vi "VectorCased.vi"(11 "XYUVArray":dbl[][](array[numeric])=[[-138.0, 28.0, -5.0, -3.0], [-92.0, 28.0, -10.0, -5.5], [-46.0, 28.0, -5.0, -10.5], [0.0, 28.0, -9.0, 3.5], [46.0, 28.0, -22.0, 1.0], [92.0, 28.0, -24.5, -9.0], [138.0, 28.0, -16.0, -23.0], [-138.0, 60.0, -6.0, -2.0], [-92.0, 60.0, -7.0, -12.0], [-46.0, 60.0, -6.0, -11.0], [0.0, 60.0, -9.0, 3.0], [46.0, 60.0, -5.5, 6.0], [92.0, 60.0, -10.0, -7.5], [138.0, 60.0, -17.0, -22.0], [-138.0, 92.0, 0.5, 2.0], [-92.0, 92.0, -1.5, -15.0], [-46.0, 92.0, -1.5, -10.5], [0.0, 92.0, 1.0, -1.5], [46.0, 92.0, 1.0, 3.0], [92.0, 92.0, -2.5, -7.5], [138.0, 92.0, -5.0, -17.0], [-138.0, 124.0, 18.5, 15.0], [-92.0, 124.0, 10.5, -2.5], [-46.0, 124.0, 6.5, -2.0], [0.0, 124.0, 7.5, 5.0], [46.0, 124.0, 9.5, 12.5], [92.0, 124.0, 14.0, 8.5], [138.0, 124.0, 6.5, -4.0], [-138.0, 156.0, 13.5, 14.5], [-92.0, 156.0, 19.5, 4.0], [-46.0, 156.0, 12.5, -1.0], [0.0, 156.0, 10.5, 3.5], [46.0, 156.0, 14.0, 11.0], [92.0, 156.0, 17.5, 10.5], [138.0, 156.0, 12.0, -4.5], [-138.0, 188.0, 9.0, 16.5], [-92.0, 188.0, 10.0, 8.0], [-46.0, 188.0, 14.0, 4.0], [0.0, 188.0, 15.5, 8.0], [46.0, 188.0, 14.5, 11.0], [92.0, 188.0, 21.5, 11.0], [138.0, 188.0, 19.0, 0.5], [-138.0, 214.0, 12.5, 11.5], [-92.0, 214.0, 17.5, 6.0], [-46.0, 214.0, 17.0, 9.5], [0.0, 214.0, 14.5, 10.5], [46.0, 214.0, 19.0, 10.5], [92.0, 214.0, 20.0, 7.0], [138.0, 214.0, 16.5, 7.0]]) -> ()   [LabVIEW 2010]
panel:
  in  "ArrowScale":dbl(slide)=0.3 min=0.0 step=0.1 scale=0.0..0.5
  in  "stop":bool
  in  "Border":dbl(slide)=0.2 min=0.0 step=0.05 scale=0.0..0.2
  in  "VectorScale":dbl(slide)=1.5 min=0.0 step=0.25 scale=0.0..10.0
  out "VectorPicture":picture
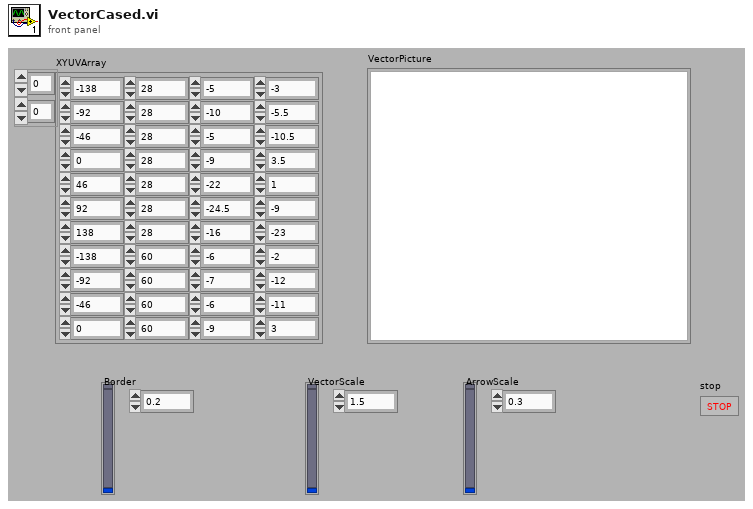
[diagram p1: front panel]
types:
  T1 = typedef "LVBoundsTypeDef.ctl" = cluster{"Width":u32, "Height":u32}
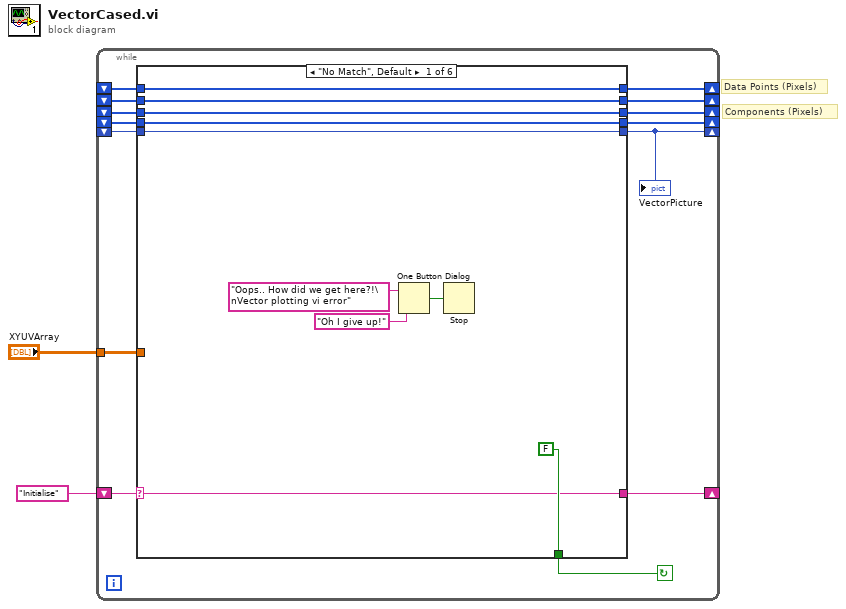
[diagram p0: block diagram]
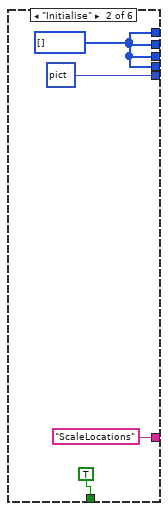
[diagram p2: hidden frame]
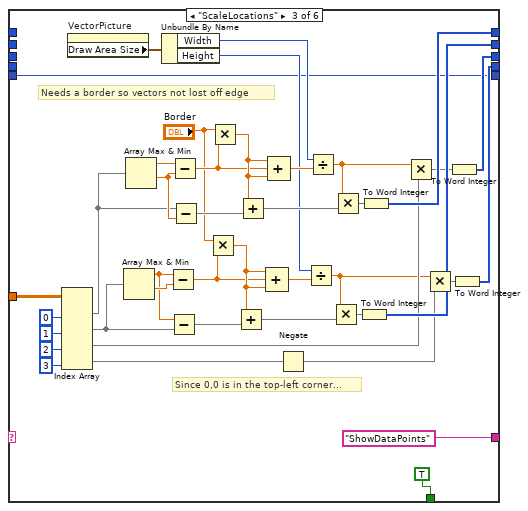
[diagram p3: hidden frame]
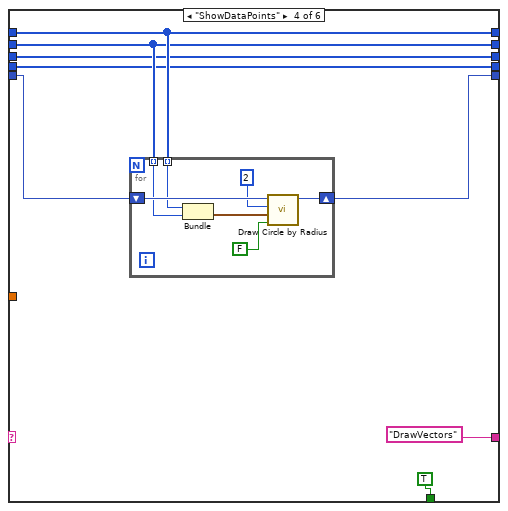
[diagram p4: hidden frame]
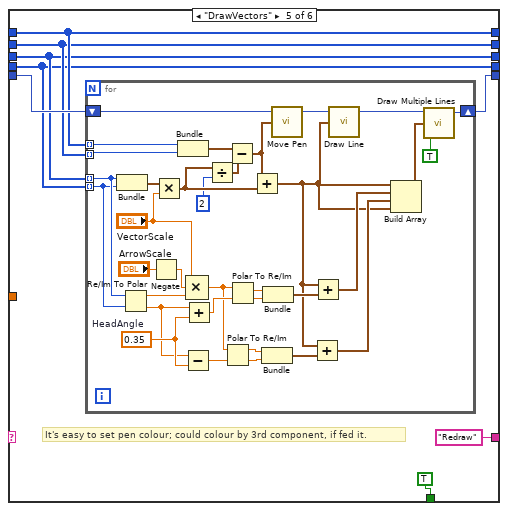
[diagram p5: hidden frame]
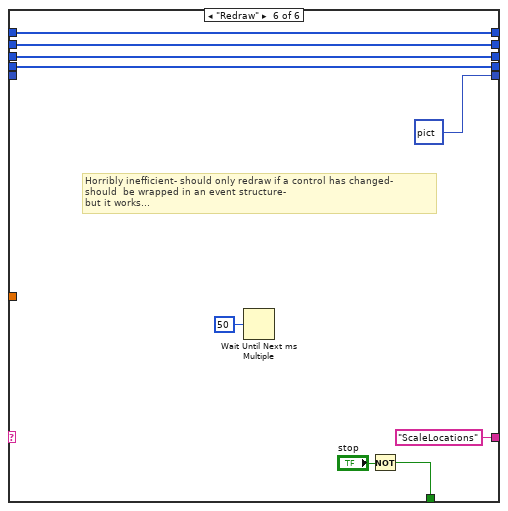
[diagram p6: hidden frame]
diagram:
  # "Components (Pixels)"
  # "Data Points (Pixels)"
  n1 = while {
    shift-right: [w12] -> _
    shift-left: "Initialise" -> [w16]
    shift-right: [w7] -> _
    shift-left: _ -> [w14]
    tunnel: "XYUVArray" -> [w13]
    shift-right: [w11] -> _
    shift-left: _ -> [w9]
    shift-right: [w10] -> _
    shift-left: _ -> [w8]
    shift-right: [w6] -> _
    shift-left: _ -> [w4]
    shift-right: [w5] -> _
    shift-left: _ -> [w3]
    stop <- w15 continue-if-true
    n2 = case shown="\"No Match\", Default" w16 {
      selector: w16 -> [w25 _ _ _ _ _]
      tunnel: [FALSE TRUE TRUE TRUE TRUE w131] -> w15
      tunnel: [w24 picture data[5B] ("new picture") w31 w75 w93 picture data[5B] ("new picture")] -> w7
      tunnel: w14 -> [w24 _ w31 w79 w94 _]
      tunnel: w13 -> [_ _ w66 _ _ _]
      tunnel: [w25 "ScaleLocations" "ShowDataPoints" "DrawVectors" "Redraw" "ScaleLocations"] -> w12
      tunnel: [w23 w27 w45 w78 w92 w137] -> w11
      tunnel: [w22 w27 w44 w77 w91 w136] -> w10
      tunnel: w9 -> [w23 _ _ w78 w92 w137]
      tunnel: w8 -> [w22 _ _ w77 w91 w136]
      tunnel: [w21 w27 w34 w74 w90 w135] -> w6
      tunnel: [w20 w27 w33 w73 w89 w134] -> w5
      tunnel: w4 -> [w21 _ _ w74 w90 w135]
      tunnel: w3 -> [w20 _ _ w73 w89 w134]
      frame "No Match", Default {
        n3 = One Button Dialog(message="Oops.. How did we get here?!\nVector plotting vi error", button name ("OK")="Oh I give up!") -> (true=w17:bool)
        n4 = Stop(stop? (T)=w17) -> ()
      }
      frame "Initialise" {
        w27 = i16[] []
      }
      frame "ScaleLocations" {
        # "Needs a border so vectors not lost off edge"
        # "Since 0,0 is in the top-left corner..."
        n5 = Index Array(array=w66, index (col) #1=0 ("disabled index (col)"), index (col) #2=1 ("index (col)"), index (col) #3=2 ("index (col)"), index (col) #4=3 ("index (col)")) -> (element #1=w64:dbl[], element #2=w50:dbl[], element #3=w40:dbl[], element #4=w36:dbl[])  [unwired: 4 in]
        n6 = property on="VectorPicture" class="Pict"() -> ("Draw Area Size"=w43:T1)  [unwired: 2 in, 2 out]
        n7 = Array Max & Min(array=w50) -> (max value=w51:dbl, min value=w55:dbl)  [unwired: 2 out]
        n8 = Array Max & Min(array=w64) -> (max value=w71:dbl, min value=w65:dbl)  [unwired: 2 out]
        n9 = Unbundle By Name(w43) -> ("Width"=w42:u32, "Height"=w41:u32)
        n10 = Subtract(x=w51, y=w55) -> (x-y=w52:dbl)
        n11 = Subtract(x=w51, y=w50) -> (x-y=w56:dbl[])
        n12 = Subtract(x=w71, y=w65) -> (x-y=w54:dbl)
        n13 = Subtract(x=w64, y=w65) -> (x-y=w63:dbl[])
        n14 = Multiply(x="Border", y=w52) -> (x*y=w57:dbl)
        n15 = Multiply(x="Border", y=w54) -> (x*y=w62:dbl)
        n16 = Add(x=w57, y=w56) -> (x+y=w59:dbl[])
        n17 = Add(x=w62, y=w63) -> (x+y=w60:dbl[])
        n18 = Compound Arithmetic op=ADD(w57, w52, w57) -> (w58:dbl)
        n19 = Compound Arithmetic op=ADD(w62, w54, w62) -> (w61:dbl)
        n20 = Negate(x=w36) -> (-x=w32:dbl[])
        n21 = Divide(x=w41, y=w58) -> (x/y=w37:dbl)
        n22 = Divide(x=w42, y=w61) -> (x/y=w39:dbl)
        n23 = Multiply(x=w37, y=w59) -> (x*y=w46:dbl[])
        n24 = Multiply(x=w39, y=w60) -> (x*y=w47:dbl[])
        n25 = To Word Integer(number=w46) -> (16bit integer=w44:i16[])
        n26 = To Word Integer(number=w47) -> (16bit integer=w45:i16[])
        n27 = Multiply(x=w39, y=w40) -> (x*y=w38:dbl[])
        n28 = Multiply(x=w37, y=w32) -> (x*y=w35:dbl[])
        n29 = To Word Integer(number=w38) -> (16bit integer=w34:i16[])
        n30 = To Word Integer(number=w35) -> (16bit integer=w33:i16[])
      }
      frame "ShowDataPoints" {
        n31 = for {
          tunnel: w78 -> [w81] mode=indexing
          tunnel: w77 -> [w80] mode=indexing
          shift-right: [w86] -> w75
          shift-left: w79 -> [w84]
          n32 = Bundle(w81, w80) -> (w82:cluster{i16, i16})  [unwired: 1 in]
          n33 = call <vilib>:"Draw Circle by Radius.vi"("fill?(F)"=FALSE, "pixel center"=w82, "radius"=i16 2, "picture"=w84) -> ("new picture"=w86:picture)  [unwired: 7 in]
        }
      }
      frame "DrawVectors" {
        # "It's easy to set pen colour; could colour by 3rd component, if fed it."
        n34 = for {
          tunnel: w90 -> [w118] mode=indexing
          tunnel: w89 -> [w117] mode=indexing
          tunnel: w92 -> [w127] mode=indexing
          tunnel: w91 -> [w126] mode=indexing
          shift-right: [w120] -> w93
          shift-left: w94 -> [w128]
          w106 = 0.35  # HeadAngle
          n35 = Bundle(w118, w117) -> (w121:cluster{i16, i16})  [unwired: 1 in]
          n36 = Re/Im To Polar(2:w117, 3:w118) -> (0:w105:dbl, 1:w112:dbl)
          n37 = Negate(x="ArrowScale") -> (-x=w96:dbl)
          n38 = Multiply(x=w121, y="VectorScale") -> (x*y=w125:cluster{dbl, dbl})
          n39 = Bundle(w127, w126) -> (w123:cluster{i16, i16})  [unwired: 1 in]
          n40 = Subtract(x=w105, y=w106) -> (x-y=w102:dbl)
          n41 = Add(x=w105, y=w106) -> (x+y=w113:dbl)
          n42 = Compound Arithmetic op=MULTIPLY("VectorScale", w96, w112) -> (w101:dbl)
          n43 = Divide(x=w125, y=2) -> (x/y=w122:cluster{dbl, dbl})
          n44 = Polar To Re/Im(2:w102, 3:w101) -> (0:w104:dbl, 1:w103:dbl)
          n45 = Subtract(x=w123, y=w122) -> (x-y=w110:cluster{dbl, dbl})
          n46 = Polar To Re/Im(2:w113, 3:w101) -> (0:w115:dbl, 1:w116:dbl)
          n47 = Add(x=w110, y=w125) -> (x+y=w97:cluster{dbl, dbl})
          n48 = Bundle(w103, w104) -> (w100:cluster{dbl, dbl})  [unwired: 1 in]
          n49 = Bundle(w116, w115) -> (w114:cluster{dbl, dbl})  [unwired: 1 in]
          n50 = call <vilib>:"Move Pen.vi"("new position"=w110, "picture"=w128) -> ("new picture"=w108:picture)  [unwired: 3 in]
          n51 = Add(x=w97, y=w100) -> (x+y=w98:cluster{dbl, dbl})
          n52 = Add(x=w97, y=w114) -> (x+y=w99:cluster{dbl, dbl})
          n53 = call <vilib>:"Draw Line.vi"("picture"=w108, "end point"=w97) -> ("new picture"=w107:picture)  [unwired: 7 in]
          n54 = Build Array(w97, w99, w98, w97) -> (w119:cluster{dbl, dbl}[])
          n55 = call <vilib>:"Draw Multiple Lines.vi"("picture"=w107, "line endpoints"=w119, "fill?(F)"=TRUE) -> ("new picture"=w120:picture)  [unwired: 6 in]
        }
      }
      frame "Redraw" {
        # "Horribly inefficient- should only redraw if a control has changed-\nshould  be wrapped in an event structure-\nbut it works..."
        n56 = Wait Until Next ms Multiple(millisecond multiple=u32 50) -> ()  [unwired: 1 out]
        n57 = Not(x="stop") -> (.not. x?=w131:bool)
      }
    }
    "VectorPicture" <- w7
  }
